vi "Shared Variable Project Filename--Const.vi"() -> (3 "Shared Variables Project Filename":string="DTACQ - Network Enabled Device Driver.lvlib")   [LabVIEW 2017, in "Shared Variables Library.lvlib"]
doc: "The filename of the main project, containing the shared variable container library."
uses:
  Shared Variables Library.lvlib
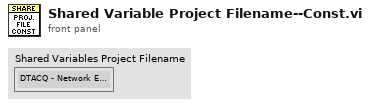
[diagram p1: front panel]
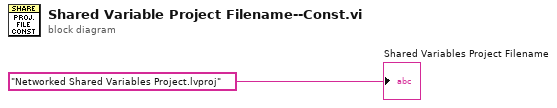
[diagram p0: block diagram]
diagram:
  "Shared Variables Project Filename" <- "Networked Shared Variables Project.lvproj"
